vi "PSAClose.vi"(8 "error in (no error)":errorcluster, 11 "PSA In":refnum<visa-resource-name>) -> (0 "error out":errorcluster)   [LabVIEW 2014]
uses:
  Agilent ESA PSA Series.lvlib
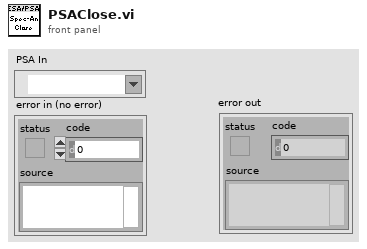
[diagram p1: front panel]
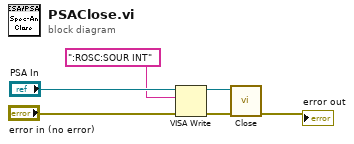
[diagram p0: block diagram]
diagram:
  n1 = VISA Write(VISA resource name="PSA In", write buffer=":ROSC:SOUR INT") -> (VISA resource name out=w2:refnum<visa-resource-name>)  [unwired: 1 in, 2 out]
  n2 = call "Close.vi"("error in (no error)"="error in (no error)", "VISA resource name"=w2) -> ("error out"=→"error out":errorcluster)  [unwired: 9 in]
